vi "JGP8three stooges.vi"() -> ()   [LabVIEW 2019]
panel:
  in  "Line & Stop":bool
  in  "Curly":bool
  in  "Larry":bool
  in  "Moe":bool
  # "Juan Gamez"
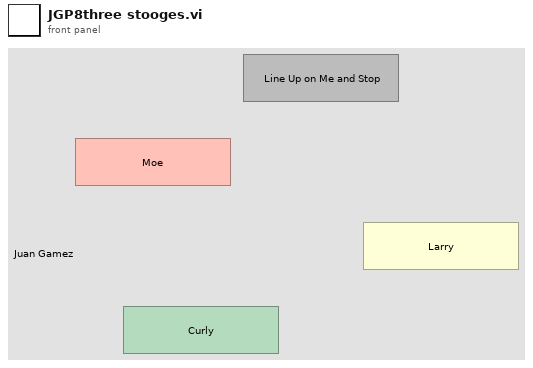
[diagram p1: front panel]
types:
  T1 = typedef "LVPositionTypeDef.ctl" = cluster{"Left":i32, "Top":i32}
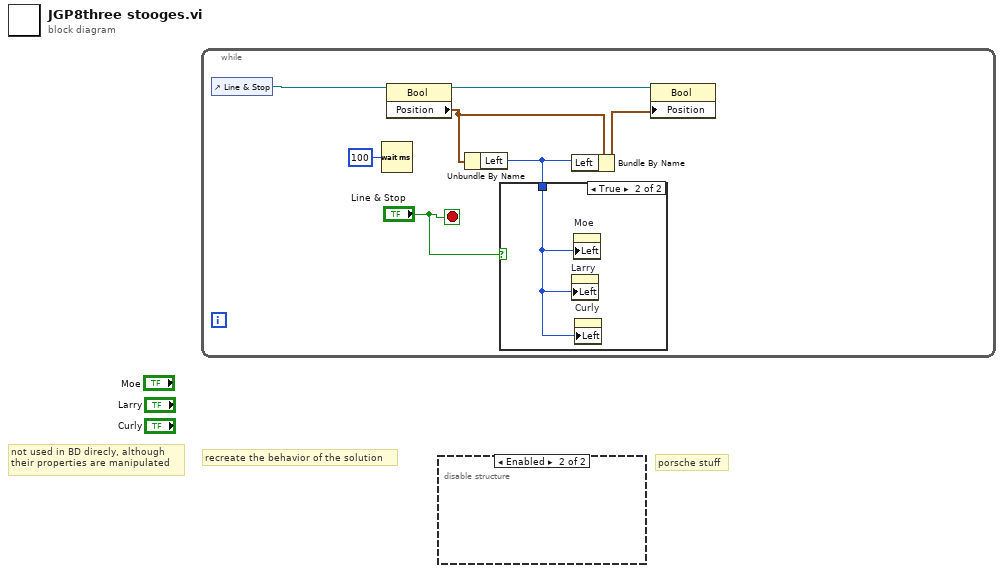
[diagram p0: block diagram]
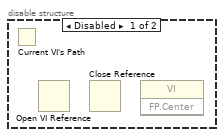
[diagram p3: hidden frame]
diagram:
  # "recreate the behavior of the solution"
  # "porsche stuff"
  # "not used in BD direcly, although \ntheir properties are manipulated"
  n1 = while {
    stop <- "Line & Stop" stop-if-true
    n2 = control-ref of="Line & Stop"() -> (w7:refnum<vi>)
    n3 = Wait (ms)(milliseconds to wait=u32 100) -> ()  [unwired: 1 out]
    n4 = property class="Bool"(reference=w7) -> (reference out=w3:refnum<vi>, "Position"=w5:T1)  [unwired: 1 in, 1 out]
    n5 = Unbundle By Name(w5) -> ("Left"=w2:i32)
    n6 = case shown="True" "Line & Stop" {
      tunnel: w2 -> [_ w8]
      frame False {
      }
      frame True {
        n7 = property on="Larry" class="Bool"("Left"=w8) -> ()  [unwired: 2 in, 2 out]
        n8 = property on="Moe" class="Bool"("Left"=w8) -> ()  [unwired: 2 in, 2 out]
        n9 = property on="Curly" class="Bool"("Left"=w8) -> ()  [unwired: 2 in, 2 out]
      }
    }
    n10 = Bundle By Name(cluster=w5, "Left"=w2) -> (w6:T1)
    n11 = property class="Bool"(reference=w3, "Position"=w6) -> ()  [unwired: 1 in, 2 out]
  }
  n12 = disable-structure shown="Enabled" {
    frame Disabled {
      n13 = Current VI's Path() -> ()  [unwired: 1 out]
      n14 = Open VI Reference() -> ()  [unwired: 6 in, 2 out]
      n15 = Close Reference() -> ()  [unwired: 2 in, 1 out]
      n16 = invoke class="VI" method="FP.Center"() -> ()  [unwired: 3 in, 3 out]
    }
    frame Enabled {
    }
  }
